vi "Distance between two filters.vi"(9 "End Filter":i32, 10 "Start Filter":i32, 11 "Wheel info":T1={"Names"=[], "Relative Position"=[0, 10000, 17000, 25000, 33000, 40000], "Wheel Name"="", "Size"=50000}) -> (1 "Moves":i32[](array[numeric]), 2 "wrap":bool, 3 "Distance":i32)   [LabVIEW 2022 SP3]
uses:
  Filter Wheel Object/Filter Wheel Details.ctl
  FW Arduino Control.lvclass
  Filter Wheel Object/Filter Wheel.lvclass
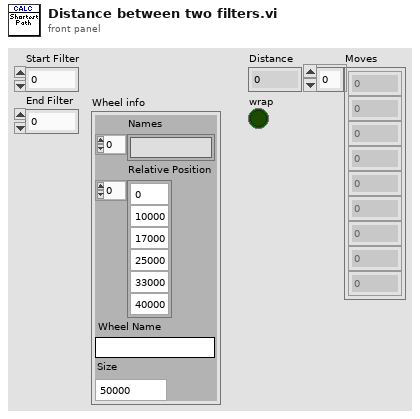
[diagram p1: front panel]
types:
  T1 = typedef "Filter Wheel.lvclass/Filter Wheel Details.ctl" = cluster{"Names":string[], "Relative Position":i32[], "Wheel Name":string, "Size":i32}
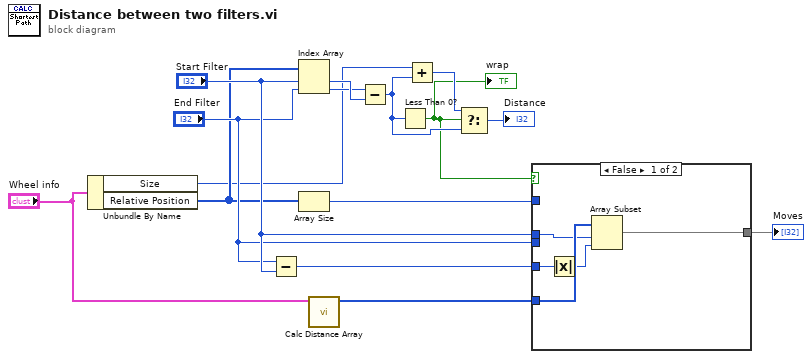
[diagram p0: block diagram]
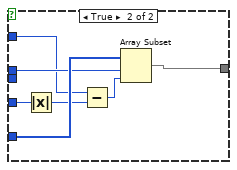
[diagram p2: hidden frame]
diagram:
  n1 = Unbundle By Name("Wheel info") -> ("Size"=w1:i32, "Relative Position"=w3:i32[])
  n2 = Subtract(x="End Filter", y="Start Filter") -> (x-y=w10:i32)
  n3 = Index Array(array=w3, index #1="Start Filter", index #2="End Filter") -> (element #1=w15:i32, element #2=w14:i32)
  n4 = Array Size(array=w3) -> (size(s)=w2:i32)
  n5 = call "Calc Distance Array.vi"("Wheel info"="Wheel info") -> ("Distances"=w4:i32[])  [unwired: 10 in]
  n6 = Subtract(x=w14, y=w15) -> (x-y=w12:i32)
  n7 = Less Than 0?(x=w12) -> (x < 0?=w6:bool)
  "wrap" <- w6
  n8 = Add(x=w1, y=w12) -> (x+y=w13:i32)
  n9 = Select(t=w13, s=w6, f=w12) -> (s? t:f=→"Distance":i32)
  n10 = case shown="False" w6 {
    tunnel: w4 -> [w20 w27]
    tunnel: "End Filter" -> [_ _]
    tunnel: w10 -> [w19 w25]
    tunnel: [w16 w24] -> w7
    tunnel: "Start Filter" -> [w17 w26]
    tunnel: w2 -> [_ w21]
    frame False {
      n11 = Absolute Value(x=w19) -> (abs(x)=w18:i32)
      n12 = Array Subset(array=w20, index=w17, length=w18) -> (w16:i32[])
    }
    frame True {
      n13 = Absolute Value(x=w25) -> (abs(x)=w23:i32)
      n14 = Subtract(x=w21, y=w23) -> (x-y=w22:i32)
      n15 = Array Subset(array=w27, index=w26, length=w22) -> (w24:i32[])
    }
  }
  "Moves" <- w7
